vi "Intersect Edge.vi"(9 "Axis Basis":i32, 10 "Contour Value":sgl, 11 "Triangle Array Cluster":cluster{"Array":sgl[], "Array 2":sgl[]}) -> (2 "In Range":bool, 3 "Intersect Point":cluster{"X":sgl, "Y":sgl, "Z":sgl})   [LabVIEW 2020, in "3D Contour.lvclass"]
uses:
  <vilib>/Math Plots/3D Math Plots/3D Contour/3D Contour/3D Contour.lvclass
panel:
  # "X Axis = 0\nY Axis = 1\nZ Axis = 2"
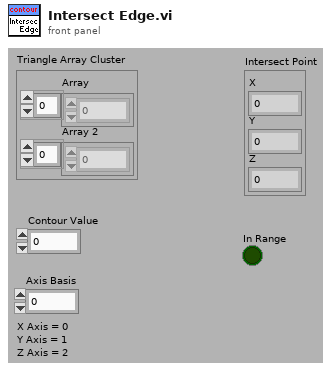
[diagram p1: front panel]
types:
  T1 = cluster{"appended array[0]":sgl, "appended array[1]":sgl, "appended array[2]":sgl}
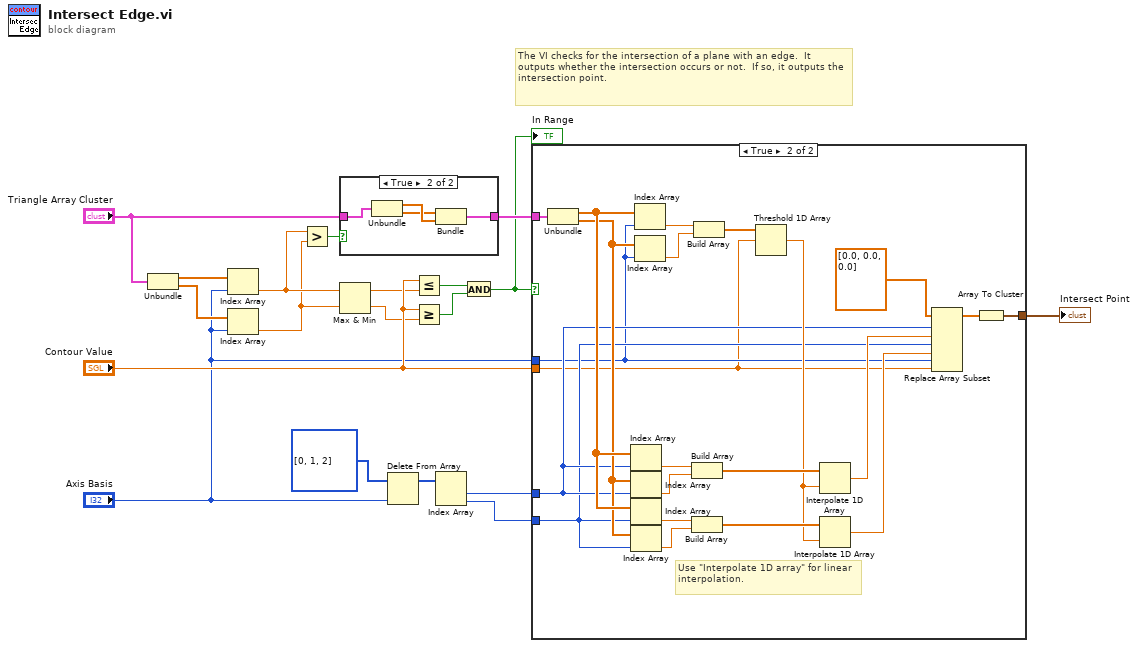
[diagram p0: block diagram]
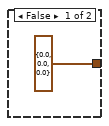
[diagram p3: hidden frame]
diagram:
  # "The VI checks for the intersection of a plane with an edge.  It outputs whether the intersection occurs or not.  If so, it outputs the intersection point."
  n1 = Unbundle("Triangle Array Cluster") -> ("Array"=w19:sgl[], "Array 2"=w18:sgl[])
  n2 = Index Array(array=w19, index="Axis Basis") -> (element=w8:sgl)
  n3 = Index Array(array=w18, index="Axis Basis") -> (element=w7:sgl)
  n4 = Greater?(x=w8, y=w7) -> (0:w13:bool)
  n5 = case shown="True" w13 {
    tunnel: "Triangle Array Cluster" -> [w20 w24]
    tunnel: [w20 w21] -> w12
    frame False {
    }
    frame True {
      n6 = Unbundle(w24) -> ("Array"=w23:sgl[], "Array 2"=w22:sgl[])
      n7 = Bundle("Array 2"=w22, "Array"=w23) -> (w21:cluster{"Array 2":sgl[], "Array":sgl[]})  [unwired: 1 out]
    }
  }
  n8 = Max & Min(x=w8, y=w7) -> (max(x,y)=w6:sgl, min(x,y)=w5:sgl)
  n9 = Delete From Array(array=i32[] [0, 1, 2], index="Axis Basis") -> (array with subset deleted=w3:i32[])  [unwired: 1 in, 1 out]
  n10 = Less Or Equal?(x="Contour Value", y=w6) -> (x <= y?=w17:bool)
  n11 = Greater Or Equal?(x="Contour Value", y=w5) -> (x >= y?=w16:bool)
  n12 = Index Array(array=w3) -> (element #1=w15:i32, element #2=w14:i32)  [unwired: 2 in]
  n13 = And(x=w17, y=w16) -> (x .and. y?=w2:bool)
  "In Range" <- w2
  n14 = case shown="True" w2 {
    tunnel: w12 -> [_ w47]
    tunnel: w15 -> [_ w32]
    tunnel: w14 -> [_ w30]
    tunnel: "Contour Value" -> [_ w26]
    tunnel: "Axis Basis" -> [_ w27]
    tunnel: [cluster{"X":sgl, "Y":sgl, "Z":sgl} {"X"=0.0, "Y"=0.0, "Z"=0.0} ("3D Point") w28] -> w9
    frame False {
    }
    frame True {
      # "Use \"Interpolate 1D array\" for linear interpolation."
      n15 = Unbundle(w47) -> ("Array 2"=w46:sgl[], "Array"=w45:sgl[])
      n16 = Index Array(array=w46, index=w32) -> (element=w44:sgl)
      n17 = Index Array(array=w45, index=w32) -> (element=w43:sgl)
      n18 = Index Array(array=w46, index=w30) -> (element=w42:sgl)
      n19 = Index Array(array=w45, index=w30) -> (element=w41:sgl)
      n20 = Index Array(array=w46, index=w27) -> (element=w40:sgl)
      n21 = Index Array(array=w45, index=w27) -> (element=w39:sgl)
      n22 = Build Array(w44, w43) -> (w38:sgl[])
      n23 = Build Array(w42, w41) -> (w36:sgl[])
      n24 = Build Array(w40, w39) -> (w37:sgl[])
      n25 = Threshold 1D Array(2:w26, 3:w37) -> (0:w35:sgl)  [unwired: 1 out]
      n26 = Interpolate 1D Array(1:w35, 2:w38) -> (0:w33:sgl)
      n27 = Interpolate 1D Array(1:w35, 2:w36) -> (0:w31:sgl)
      n28 = Replace Array Subset(array=sgl[] [0.0, 0.0, 0.0] ("appended array"), new element #1=w33, index #1=w32, new element #2=w31, index #2=w30, new element #3=w26, index #3=w27) -> (w29:sgl[])
      n29 = Array To Cluster(array=w29) -> (cluster=w28:T1)
    }
  }
  "Intersect Point" <- w9
